vi "Get configuration chain.vi"(8 "error in (no error)":errorcluster, 11 "AutofocusBase in":refnum<class "Autofocus.lvclass">) -> (0 "error out":errorcluster, 1 "class name":string[](array[string]), 2 "configuration chain":variant[](array[variant]), 3 "AutofocusBase out":refnum<class "Autofocus.lvclass">)   [LabVIEW 2012, in "Autofocus.lvclass"]
doc: "Returns an array of variants containing the configuration clusters of each class in the inheritance chain (lowest child class first), together with an array of all class names in the inheritance chain.\n\nFor classes without configuration cluster, the configuration chain contains empty variants."
uses:
  Autofocus.lvclass
  <vilib>/Distrio/Murmex/Murmex/Murmex.lvclass
  Autofocus.lvclass/Autofocus.ctl
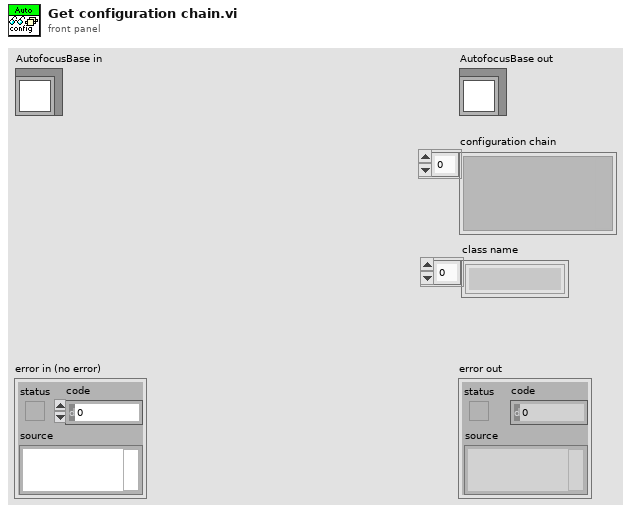
[diagram p1: front panel]
types:
  T1 = typedef "Autofocus.lvclass/configuration cluster.ctl" = cluster{"Camera component name":string, "Stages component name":string, "Tomo component name":string, "Epsilon (HC)":dbl, "Epsilon (GS)":dbl, "Number of subregions":T2}
  T2 = typedef "Autofocus.lvclass/number of subregions.ctl" = i32
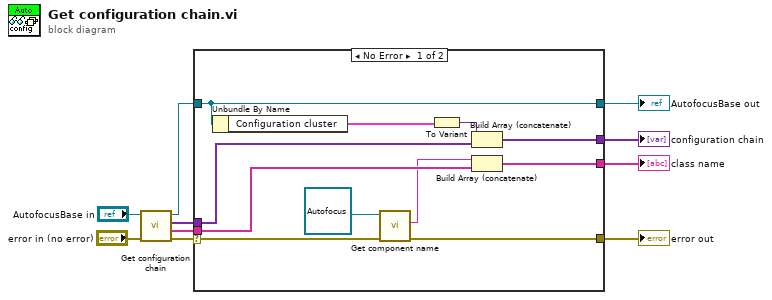
[diagram p0: block diagram]
diagram:
  n1 = call-parent "Get configuration chain.vi"("error in (no error)"="error in (no error)", "MurmexBase in"="AutofocusBase in") -> ("error out"=w8:errorcluster, "class name"=w6:string[], "configuration chain"=w5:variant[], "MurmexBase out"=w4:refnum<class "Autofocus.lvclass">)  [unwired: 6 in]
  n2 = case shown="No Error" w8 {
    selector: w8 -> [w21 w22]
    tunnel: [w20 w22] -> w7
    tunnel: w6 -> [w13 _]
    tunnel: w5 -> [w14 _]
    tunnel: w4 -> [w18 w23]
    tunnel: [w18 w23] -> w3
    tunnel: [w11 _] -> w2
    tunnel: [w15 _] -> w1
    frame No Error {
      n3 = Unbundle By Name(w18) -> ("Configuration cluster"=w16:T1)
      n4 = call <vilib>:"Get component name.vi"("error in (no error)"=w21, "Murmex in"=refnum<class "Autofocus.lvclass"> refnum ("Autofocus.lvclass")) -> ("error out"=w20:errorcluster, "component name"=w12:string)  [unwired: 7 in, 1 out]
      n5 = To Variant(anything=w16) -> (Variant=w17:variant)
      n6 = Build Array (concatenate)(w17, w14) -> (w15:variant[])
      n7 = Build Array (concatenate)(w12, w13) -> (w11:string[])
    }
    frame Error {
    }
  }
  "error out" <- w7
  "AutofocusBase out" <- w3
  "configuration chain" <- w1
  "class name" <- w2
